vi "Robot Global Data.vi"() -> ()   [LabVIEW 2014]
doc: "This global VI can contain as many global variables as you need. Place a control on the panel, give it a good name. To read or write to it from a VI, drag the icon to the diagram of that VI. You can also drag from the project. Click on the node to change which global you access. You shouldn't have multiple locations writing to a global or it will cause a race-condition."
uses:
  <vilib>/Rock Robotics/WPI/Camera/WPI_CameraImageSize.ctl
  <vilib>/Rock Robotics/WPI/DriverStation/WPI_DriverStationRobotMode2.ctl
panel:
  out "Odometer- Elevator":dbl
  in  "Auto intake":bool
  in  "In position":bool
  out "Drivetrain state auto":T1(ring)
  out "Chutador state":T2(ring)
  in  "Carrying bin":bool
  in  "Po larga josney":bool
  out "Elevator mode - auto":T3(ring)
  in  "Bin in?":bool
  out "Elevator mode":T4(ring)
  out "Left Wheel":dbl
  out "Right Wheel":dbl
  out "Chutador Analog":dbl
  in  "Chutador Volta":bool
  in  "Intake override":dbl
  in  "Manual Load":bool
  in  "Solenoide":bool
  in  "Release":bool
  in  "Get knocked Bin":bool
  in  "Get Bin":bool
  in  "Get Tote":bool
  out "Elevator Target":dbl
  out "Elevator Rate":dbl
  out "Intake Speed":dbl
  in  "Gripper State":bool
  in  "Intake Enabled?":bool
  out "Elevator position":dbl
  in  "Elevator Down?":bool
  in  "Elevator Up?":bool
  in  "Tote in?":bool
  in  "Switch Chutador":bool
  in  "Chutador":bool
  in  "Robot Mode":T5
  in  "image size":T6=enum."320x240"
  in  "Enable Vision":bool
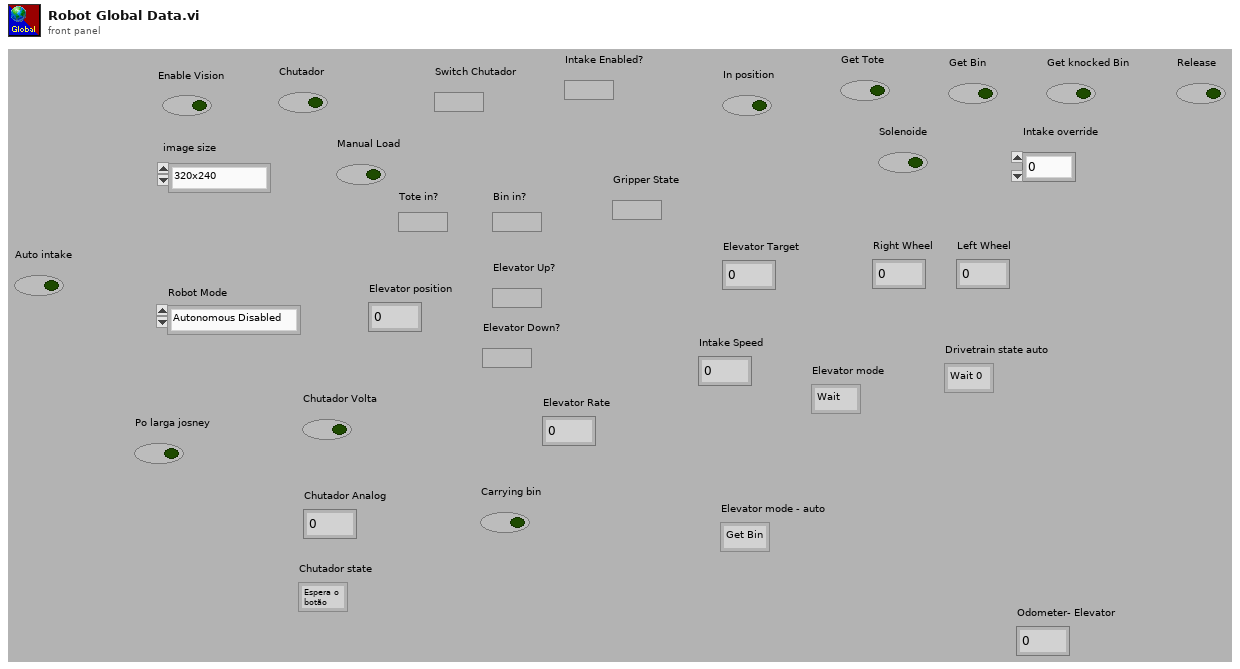
[diagram p1: front panel]
types:
  T1 = enum16{"Wait 0", "Reta 1", "Wait 1", "Reta 2", "Wait 2", "Curva 1", "Wait 3", "Reta 3", "Curva 2", "Wait 4", "Reta 4"}
  T2 = enum16{"Espera o botão", "Bate", "Para", "Volta", ""}
  T3 = enum16{"Get Bin", "Get Tote", "Wait 1", "Release"}
  T4 = enum16{"Wait", "Empty state", "Get Bin", "Get Tote First", "Get Knocked Bin", "Close Gripper - Bin", "Close Gripper", "Carry Bin Mode", "Carry Tote Mode", "Get Tote", "Change Height", "Open Gripper", "Get to 0", "Release Pile"}
  T5 = typedef "WPI_DriverStationRobotMode2.ctl" = enum16{"Autonomous Disabled", "Autonomous Enabled", "Teleop Disabled", "Teleop Enabled", "Disconnected", "Finish", "Test Disabled", "Test Enabled", "Emergency Stopped"}
  T6 = typedef "WPI_CameraImageSize.ctl" = enum16{"640x480", "320x240", "160x120", "Custom"}
diagram:
